vi "Chronos TDMS Viewer Generate XY Graph.vi"(8 "error in (no error)":errorcluster, 11 "Limit Plot Map":T1) -> (0 "error out":errorcluster, 3 "XY Graph":cluster{dbl[], dbl[]}[](graph))   [LabVIEW 2021]
uses:
  GUI/Chronos cluster Map Limit Plots.ctl
  typedefs/Chronos cluster Plot Data and Limits.ctl
  cluster CC Channel from TDMS.ctl
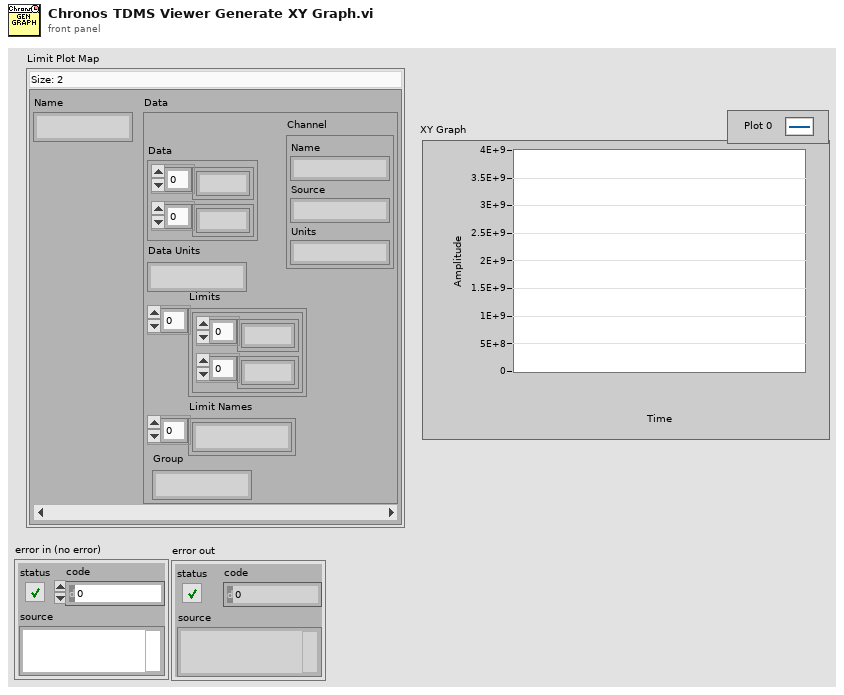
[diagram p1: front panel]
types:
  T1 = typedef "Chronos cluster Map Limit Plots.ctl" = map{string, T2}
  T2 = typedef "Chronos cluster Plot Data and Limits.ctl" = cluster{"Data":cluster{dbl[], dbl[]}, "Data Units":string, "Limits":cluster{dbl[], dbl[]}[], "Limit Names":string[], "Channel":T3, "Group":string}
  T3 = typedef "cluster CC Channel from TDMS.ctl" = cluster{"Name":string, "Source":string, "Units":string}
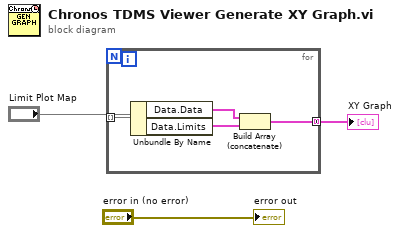
[diagram p0: block diagram]
diagram:
  n1 = for {
    tunnel: "Limit Plot Map" -> [w7] mode=indexing
    tunnel: [w4] -> w2 mode=concatenating
    n2 = Unbundle By Name(w7) -> ("Data.Data"=w6:cluster{dbl[], dbl[]}, "Data.Limits"=w5:cluster{dbl[], dbl[]}[])
    n3 = Build Array (concatenate)(w6, w5) -> (w4:cluster{dbl[], dbl[]}[])
  }
  "XY Graph" <- w2
  "error out" <- "error in (no error)"
